vi "PASCO_PID.vi"(0 "Delta":dbl(slide) scale=0.0..1.0, 9 "Integral Reset":bool, 11 "Deadband":dbl=0.001, 12 "P Gain":dbl=1.0, 13 "I Gain":dbl, 14 "D Gain":dbl) -> (4 "Output":dbl, 10 "IsThere":bool)   [LabVIEW 2014]
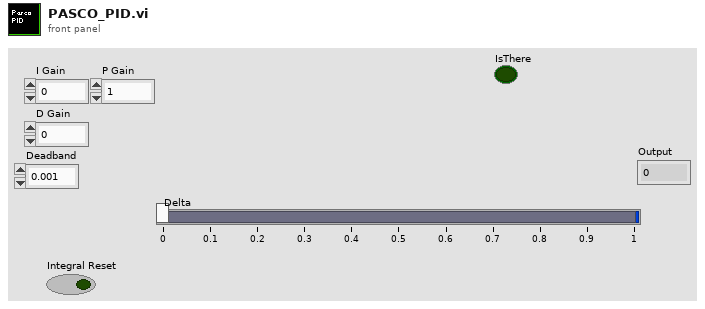
[diagram p1: front panel]
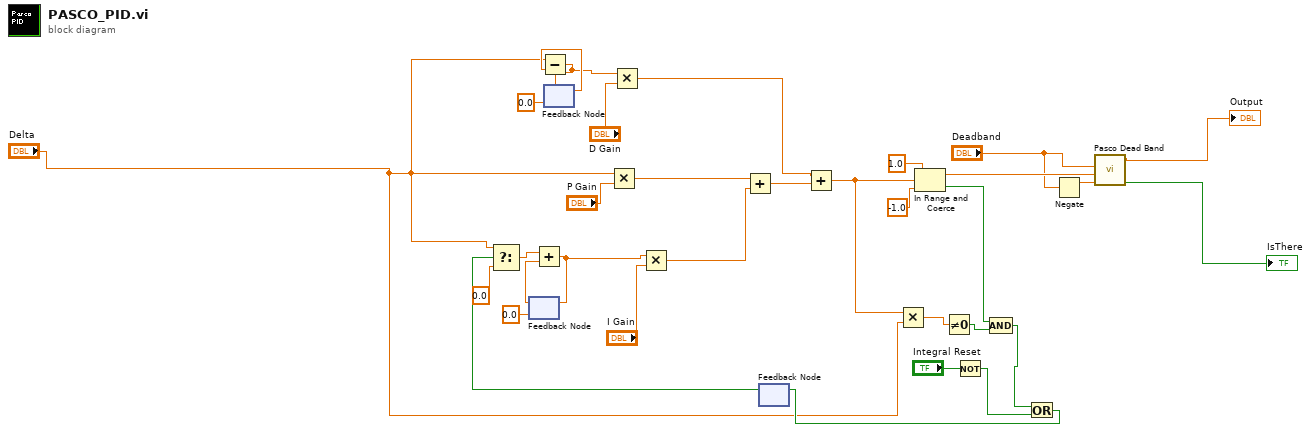
[diagram p0: block diagram]
diagram:
  n1 = feedback #1(0.0) -> (w29:dbl)
  n2 = feedback #2(0.0) -> (w28:dbl)
  n3 = Subtract(x="Delta", y=w28) -> (x-y=w27:dbl)
  n4 = feedback-in #2(w27) -> ()
  n5 = Multiply(x="Delta", y="P Gain") -> (x*y=w11:dbl)
  n6 = Multiply(x=w27, y="D Gain") -> (x*y=w20:dbl)
  n7 = feedback #3() -> (w14:bool)  [unwired: 1 in]
  n8 = Select(t="Delta", s=w14, f=0.0) -> (s? t:f=w21:dbl)
  n9 = Add(x=w21, y=w29) -> (x+y=w12:dbl)
  n10 = feedback-in #1(w12) -> ()
  n11 = Multiply(x=w12, y="I Gain") -> (x*y=w10:dbl)
  n12 = Add(x=w11, y=w10) -> (x+y=w19:dbl)
  n13 = Add(x=w20, y=w19) -> (x+y=w18:dbl)
  n14 = Multiply(x=w18, y="Delta") -> (x*y=w25:dbl)
  n15 = In Range and Coerce(upper limit=1.0, x=w18, lower limit=-1.0) -> (coerced(x)=w17:dbl, In Range?=w23:bool)
  n16 = Not Equal To 0?(x=w25) -> (x != 0?=w24:bool)
  n17 = Not(x="Integral Reset") -> (.not. x?=w7:bool)
  n18 = Compound Arithmetic op=AND(w23, w24) -> (w8:bool)
  n19 = Or(x=w8, y=w7) -> (x .or. y?=w6:bool)
  n20 = feedback-in #3(w6) -> ()
  n21 = Negate(x="Deadband") -> (-x=w16:dbl)
  n22 = call "Pasco Dead Band.vi"("lower limit"=w16, "PWM Power"=w17, "upper limit"="Deadband") -> ("Integral Reset"=→"IsThere":bool, "PWM Power"=→"Output":dbl)  [unwired: 7 in]
